vi "tunnel_simple.vi"() -> ()   [LabVIEW 2021]
uses:
  <vilib>/numeric/Random Number (Range) DBL.vi
panel:
  out "Maximum value":dbl
  out "Array":dbl[](array[numeric])
  out "Done":bool
  out "random number":dbl
  out "iteration counter":i32
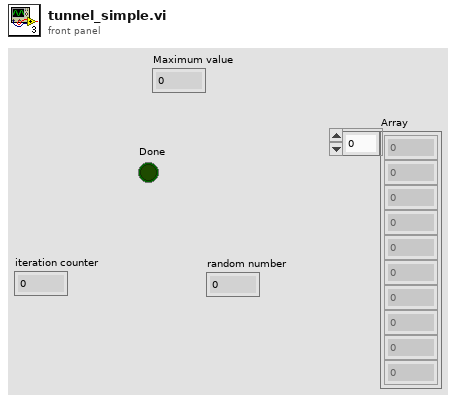
[diagram p1: front panel]
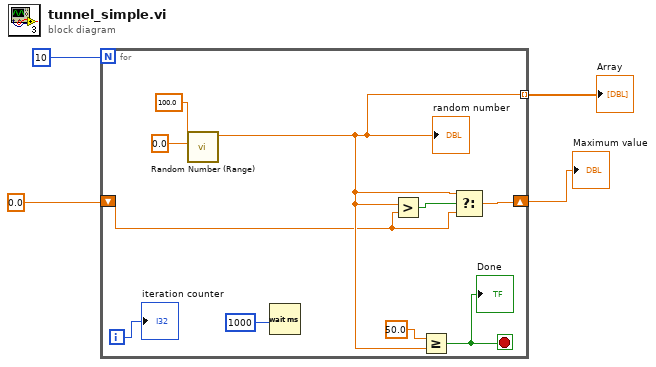
[diagram p0: block diagram]
diagram:
  n1 = for {
    N: 10 -> [_]
    tunnel: [w7] -> w3 mode=indexing
    shift-right: [w6] -> w2
    shift-left: 0.0 -> [w5]
    i -> [w12]
    stop <- w9 stop-if-true
    n2 = call-poly <vilib>:"Random Number (Range).vi"("lower bound (0)"=0.0, "upper bound (100)"=100.0) -> ("number"=w7:dbl)  [unwired: 9 in]
    "random number" <- w7
    n3 = Wait (ms)(milliseconds to wait=1000) -> ()  [unwired: 1 out]
    n4 = Greater?(x=w7, y=w5) -> (0:w8:bool)
    n5 = Greater Or Equal?(x=50.0, y=w7) -> (x >= y?=w9:bool)
    "Done" <- w9
    n6 = Select(t=w7, s=w8, f=w5) -> (s? t:f=w6:dbl)
    "iteration counter" <- w12
  }
  "Array" <- w3
  "Maximum value" <- w2
